vi "update destination folder.vi"(8 "error in":errorcluster, 11 "Picture File in":refnum<class "Picture File.lvclass">) -> (0 "error out":errorcluster, 3 "Picture File out":refnum<class "Picture File.lvclass">)   [LabVIEW 2023, in "File Classes.lvlib" / "Picture File.lvclass"]
uses:
  Picture File.lvclass
  Picture File.lvclass/Picture File.ctl
  File/File.lvclass/File.ctl
  File/Accessors/Write destination path.vi
  File/Accessors/Read scanners list.vi
  File/Accessors/Read destination path.vi
  File/Accessors/Read mode.vi
  File/File.lvclass
panel:
  # "Output Indicators"
  # "Input Controls"
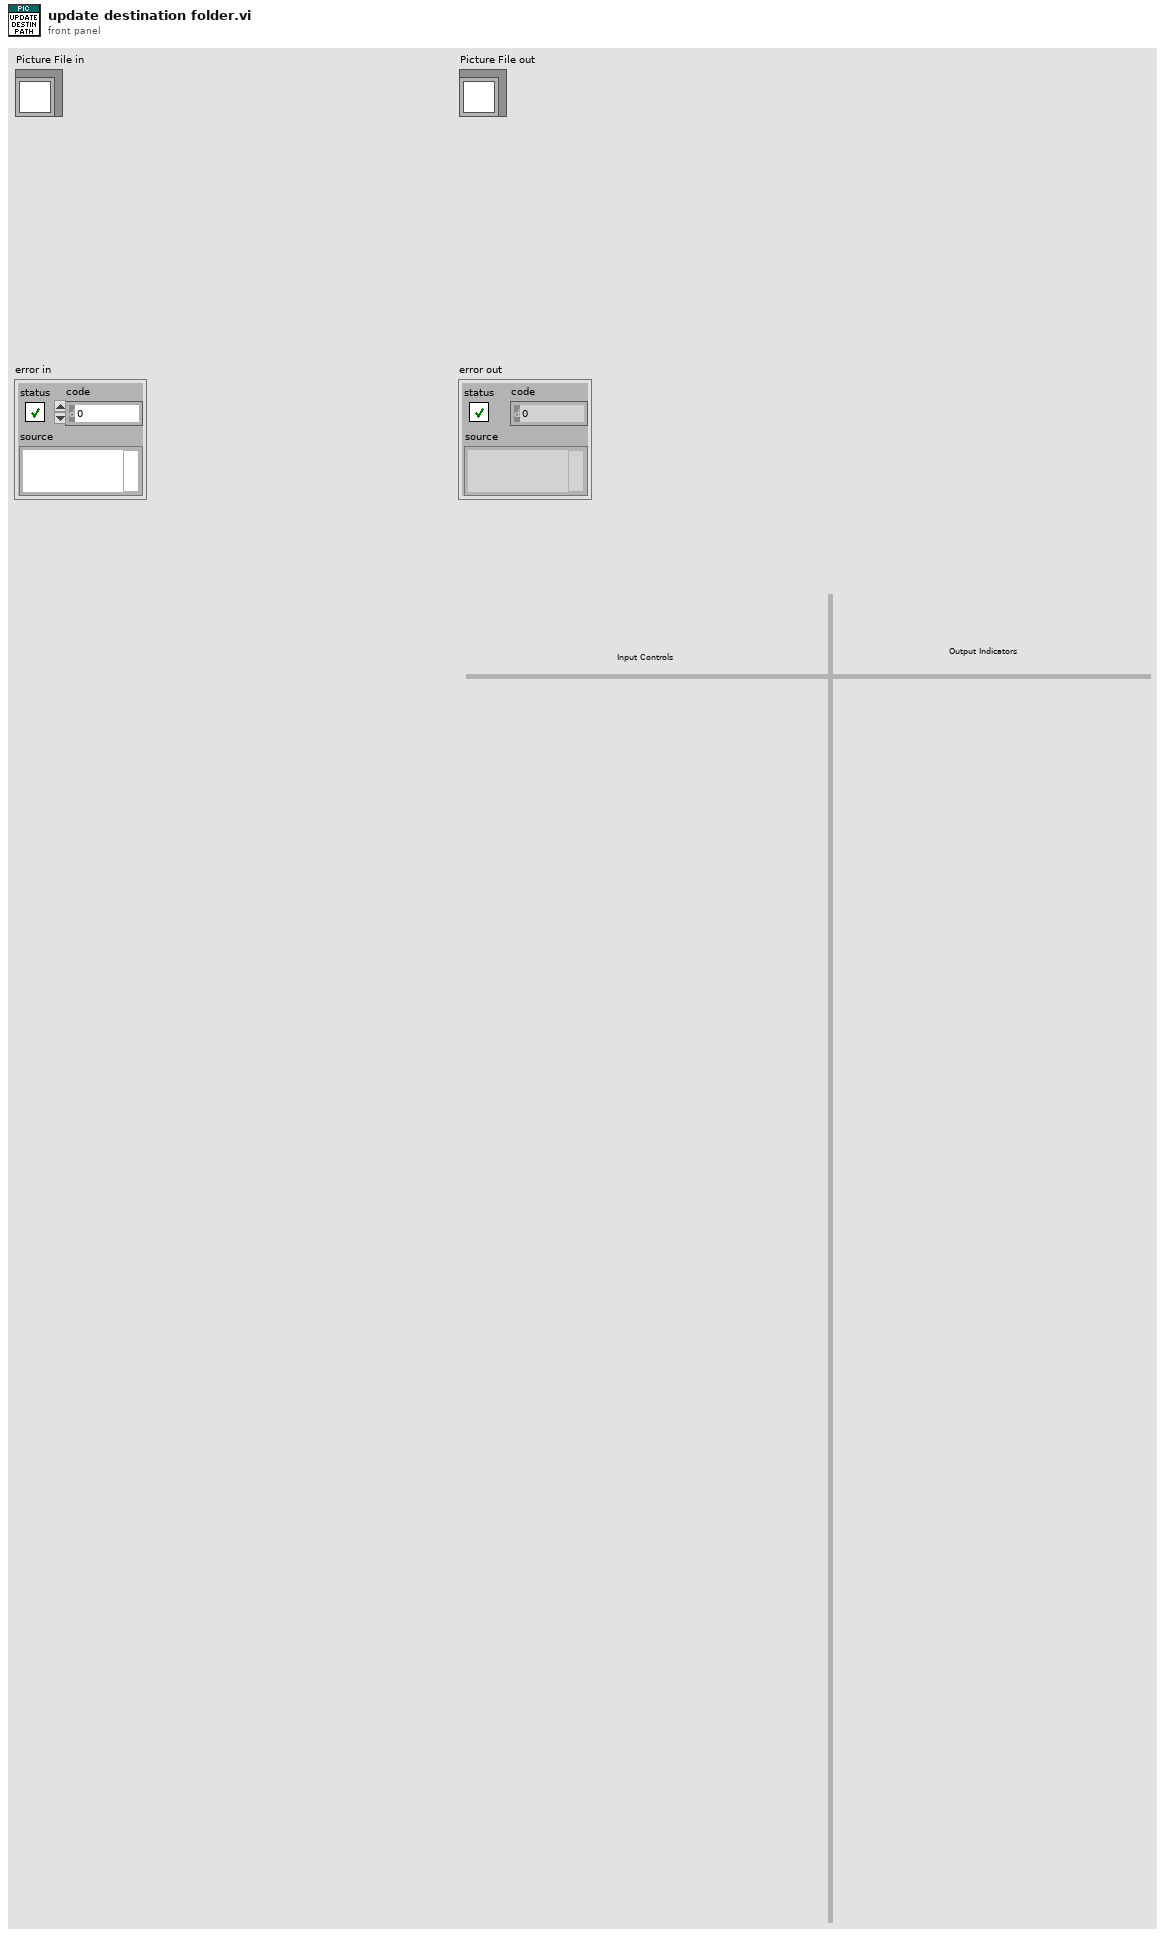
[diagram p1: front panel]
types:
  T1 = typedef "File Classes.lvlib/exif data cluster.ctl" = cluster{"Make":string, "Model":string, "Orientation":u16, "Date":timestamp, "Width":u16, "Height":u16, "Square?":bool, "File Name":string, "Extension":string, "Valid?":bool, "Path":path, "size":i64, "No Ext?":bool, "prefix?":bool, "String":string, "Name Type":T2}
  T2 = typedef "File Classes.lvlib/rename type enum.ctl" = enum16{"Date & Time (Default)", "Model Sufix", "Event Sufix", "Model & Event Sufix"}
  T3 = typedef "File Classes.lvlib/file operation settings mode.ctl" = enum16{"Copy Files", "Move Files", "Rename Files"}
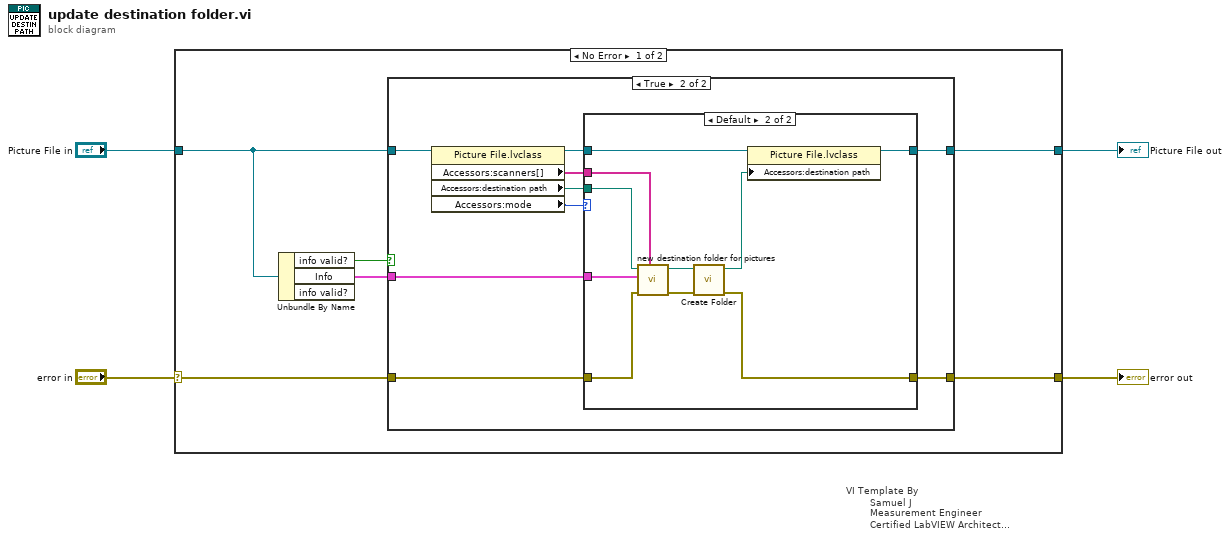
[diagram p0: block diagram]
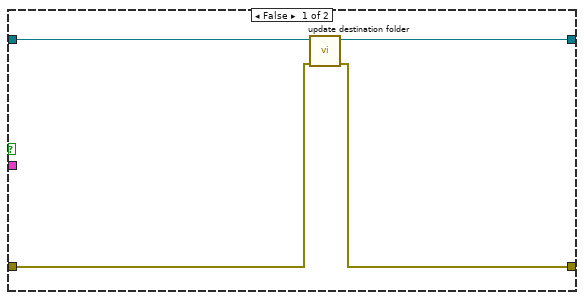
[diagram p2: hidden frame]
diagram:
  n1 = case "VI Template By\n        Samuel J\n        Measurement Engineer\n        Certified LabVIEW Architect\n        Vestas Technology R&D Chennai" shown="No Error" "error in" {
    selector: "error in" -> [w7 w37]
    tunnel: [w8 w37] -> w3
    tunnel: [w10 w36] -> w2
    tunnel: "Picture File in" -> [w9 w36]
    frame No Error {
      n2 = Unbundle By Name(w9) -> ("info valid?"=w6:bool, "Info"=w5:T1)  [unwired: 1 out]
      n3 = case shown="True" w6 {
        tunnel: [w14 w21] -> w10
        tunnel: w9 -> [w13 w23]
        tunnel: [w11 w16] -> w8
        tunnel: w7 -> [w12 w17]
        tunnel: w5 -> [_ w18]
        frame False {
          n4 = call-parent "update destination folder.vi"("error in (no error)"=w12, "File in"=w13) -> ("error out"=w11:errorcluster, "File out"=w14:refnum<class "Picture File.lvclass">)  [unwired: 8 in]
        }
        frame True {
          n5 = property class="Picture File.lvclass"(reference=w23) -> (reference out=w22:refnum<class "Picture File.lvclass">, "Accessors:scanners[]"=w19:string[], "Accessors:destination path"=w20:path, "Accessors:mode"=w15:T3)  [unwired: 1 in, 1 out]
          n6 = case shown="Default" w15 {
            tunnel: w22 -> [w25 w35]
            tunnel: [w25 w34] -> w21
            tunnel: w20 -> [_ w33]
            tunnel: w19 -> [_ w32]
            tunnel: w18 -> [_ w31]
            tunnel: w17 -> [w24 w30]
            tunnel: [w24 w26] -> w16
            frame "Rename Files" {
            }
            frame Default {
              n7 = call "new destination folder for pictures.vi"("scanners[]"=w32, "error in (no error)"=w30, "Info"=w31, "dest path"=w33) -> ("error in (no error) 2"=w27:errorcluster, "new dest filder path"=w29:path)  [unwired: 6 in]
              n8 = call <userlib>:"Create Folder.vi"("error in"=w27, "Directory Path"=w29) -> ("error out"=w26:errorcluster, "dup Directory Path"=w28:path)  [unwired: 8 in]
              n9 = property class="Picture File.lvclass"(reference=w35, "Accessors:destination path"=w28) -> (reference out=w34:refnum<class "Picture File.lvclass">)  [unwired: 1 in, 1 out]
            }
          }
        }
      }
    }
    frame Error {
    }
  }
  "error out" <- w3
  "Picture File out" <- w2
